vi "Gain Double to Int.vi"(10 "Gain Double":dbl) -> (2 "Gain Setting":u16(ring) items=["0 dB Gain"=0, "20 dB Gain"=2, "40 dB Gain"=4])   [LabVIEW 2020]
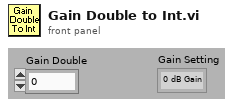
[diagram p1: front panel]
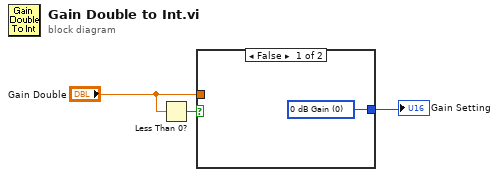
[diagram p0: block diagram]
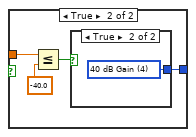
[diagram p2: hidden frame]
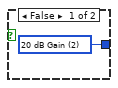
[diagram p3: hidden frame]
diagram:
  n1 = Less Than 0?(x="Gain Double") -> (x < 0?=w3:bool)
  n2 = case shown="False" w3 {
    tunnel: "Gain Double" -> [_ w8]
    tunnel: [w4 w5] -> w1
    frame False {
      w4 = u16 0 items=["0 dB Gain"=0, "20 dB Gain"=2, "40 dB Gain"=4] ("Gain Setting")
    }
    frame True {
      n3 = Less Or Equal?(x=w8, y=-40.0) -> (x <= y?=w6:bool)
      n4 = case shown="True" w6 {
        tunnel: [w9 w10] -> w5
        frame False {
          w9 = u16 2 items=["0 dB Gain"=0, "20 dB Gain"=2, "40 dB Gain"=4] ("Gain Setting")
        }
        frame True {
          w10 = u16 4 items=["0 dB Gain"=0, "20 dB Gain"=2, "40 dB Gain"=4] ("Gain Setting")
        }
      }
    }
  }
  "Gain Setting" <- w1
